vi "Append String Table To Document.vi"() -> ()   [LabVIEW 2017]
doc: "Demonstrates how to add string table to an MS Office document."
uses:
  Users/Neo/Desktop/Dev_Tools_BR/LabVIEW_NPOI/src/LabVIEW NPOI/Document/Document.lvclass/Document.ctl
  a5f45f26-4779-47fc-abe2-073284c4cecd.vi
  Users/Neo/Desktop/Dev_Tools_BR/LabVIEW_NPOI/src/LabVIEW NPOI/Document/Get FilePath.vi
  Users/Neo/Desktop/Dev_Tools_BR/LabVIEW_NPOI/src/LabVIEW NPOI/Document/Append Table (string).vi
  Users/Neo/Desktop/Dev_Tools_BR/LabVIEW_NPOI/src/LabVIEW NPOI/Document/Document.lvclass
panel:
  in  "#Columns":i32=100
  in  "#Rows":i32=2
  out "File Path":path
  in  "Document Format":enum16{"xlsx", "xls", "docx", "doc"}(ring)
  # "Overview: Demonstrates how to add string table to an MS Office document.\nInstructions:\n1. Select the Document Format you want to create.\n        Optionally: You can change the Text and the Column and Row numbers.\n2. Run the VI.\n3. The generated document will be located at the path indicated by File Path.\n4. Delete the temporary Document file when you are done."
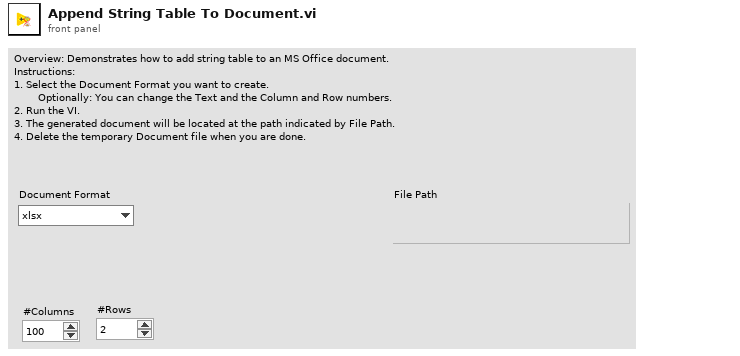
[diagram p1: front panel]
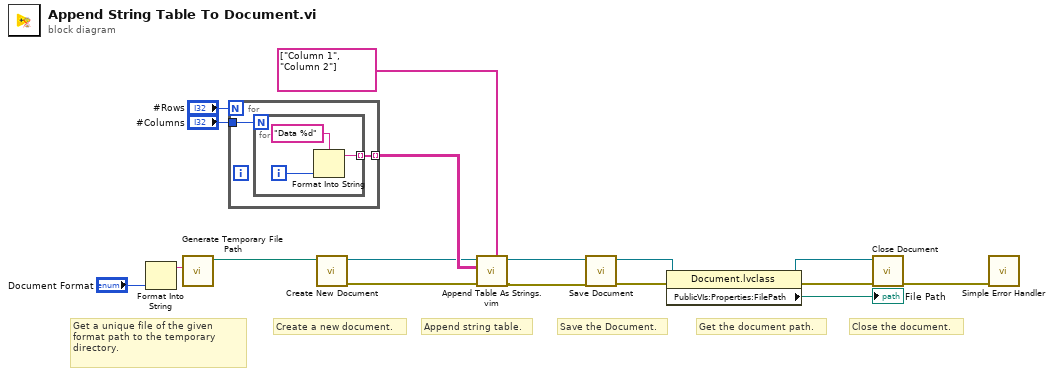
[diagram p0: block diagram]
diagram:
  # "Close the document."
  # "Get the document path."
  # "Save the Document."
  # "Append string table."
  # "Create a new document."
  # "Get a unique file of the given format path to the temporary directory."
  n1 = Format Into String("Document Format") -> (resulting string=w4:string)  [unwired: 3 in, 1 out]
  n2 = call <vilib>:"Generate Temporary File Path.vi"("Temporary File Extension (tmp)"=w4) -> ("Unique Temporary File Path"=w3:path)  [unwired: 9 in, 1 out]
  n3 = for {
    N: "#Rows" -> [_]
    tunnel: [w19] -> w6 mode=indexing
    tunnel: "#Columns" -> [w18]
    n4 = for {
      N: w18 -> [_]
      tunnel: [w22] -> w19 mode=indexing
      i -> [w20]
      n5 = Format Into String(format string="Data %d", w20) -> (resulting string=w22:string)  [unwired: 2 in, 1 out]
    }
  }
  n6 = call "Create New Document.vi"("File Path"=w3) -> ("error out"=w1:errorcluster, "Document out"=w2:refnum<class "Document.lvclass">)  [unwired: 9 in]
  n7 = call "Append Table As Strings.vim"("Column Headers"=string[] ["Column 1", "Column 2"], "error in (no error)"=w1, "Table"=w6, "Document in"=w2) -> ("error out"=w7:errorcluster, "Document out"=w8:refnum<class "Document.lvclass">)  [unwired: 6 in]
  n8 = call "Save Document.vi"("error in (no error)"=w7, "Document in"=w8) -> ("error out"=w14:errorcluster, "Document out"=w17:refnum<class "Document.lvclass">)  [unwired: 8 in]
  n9 = property class="Document.lvclass"(reference=w17, error in=w14) -> (reference out=w15:refnum<class "Document.lvclass">, error out=w13:errorcluster, "PublicVIs:Properties:FilePath"=→"File Path":path)
  n10 = call "Close Document.vi"("error in (no error)"=w13, "Document in"=w15) -> ("error out"=w16:errorcluster)  [unwired: 9 in]
  n11 = call <vilib>:"Simple Error Handler.vi"("error in (no error)"=w16) -> ()  [unwired: 4 in, 5 out]
